vi "Set Position.vi"(8 "error in (no error)":errorcluster, 9 "Increment":i32, 10 "FP Bounds":T1, 11 "LV MDI.lvclass":refnum<class "LV MDI.lvclass">) -> (0 "error out":errorcluster, 3 "LV MDI.lvclass":refnum<class "LV MDI.lvclass">)   [LabVIEW 2016, in "LV MDI.lvclass"]
uses:
  LV MDI.lvclass
  <vilib>/Utility/miscctls.llb/LVRectTypeDef.ctl
  LV MDI.lvclass/LV MDI.ctl
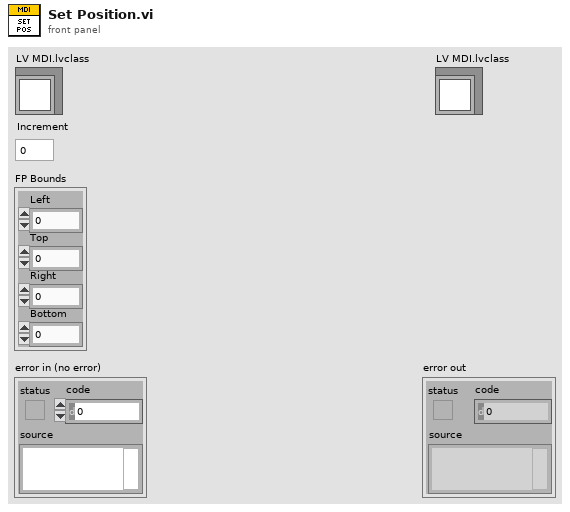
[diagram p1: front panel]
types:
  T1 = typedef "LVRectTypeDef.ctl" = cluster{"Left":i16, "Top":i16, "Right":i16, "Bottom":i16}
  T2 = cluster{"Left":i32, "Top":i32, "Right":i32, "Bottom":i32}
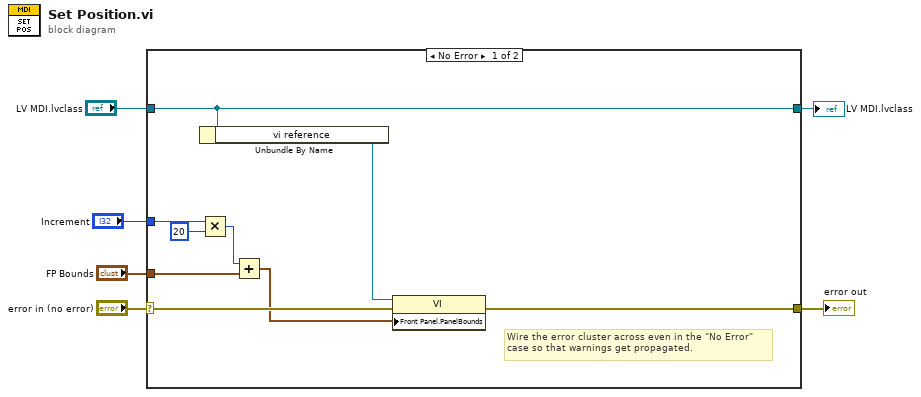
[diagram p0: block diagram]
diagram:
  n1 = case shown="No Error" "error in (no error)" {
    selector: "error in (no error)" -> [w15 w17]
    tunnel: [w14 w17] -> w5
    tunnel: [w13 w16] -> w1
    tunnel: "LV MDI.lvclass" -> [w13 w16]
    tunnel: "FP Bounds" -> [w11 _]
    tunnel: "Increment" -> [w8 _]
    frame No Error {
      # "Wire the error cluster across even in the \"No Error\"\ncase so that warnings get propagated."
      n2 = Unbundle By Name(w13) -> ("vi reference"=w12:refnum<vi>)
      n3 = Multiply(x=w8, y=20) -> (x*y=w9:i32)
      n4 = Add(x=w9, y=w11) -> (x+y=w10:T2)
      n5 = property class="VI"(reference=w12, error in=w15, "Front Panel.PanelBounds"=w10) -> (error out=w14:errorcluster)  [unwired: 1 out]
    }
    frame Error {
    }
  }
  "error out" <- w5
  "LV MDI.lvclass" <- w1
